vi "Result.Generate Xlink Overall Result.vi"(10 "Measurements":T2[](array[typedef]) {"Status" items=["LOG", "PASS", "FAIL", "ERROR"]}, 11 "Result":T4) -> (2 "PASS":bool, 3 "Measurement":T1)   [LabVIEW 2018]
uses:
  Result XML/TestResult.Symptom.ctl
  Result XML/TestResult.Symptom.State.ctl
  Result.Measurement Item.ctl
  Result.Measurement and Attribute Item Status.ctl
  Result.Factory Logix XLink Adapter, Measurement Item.ctl
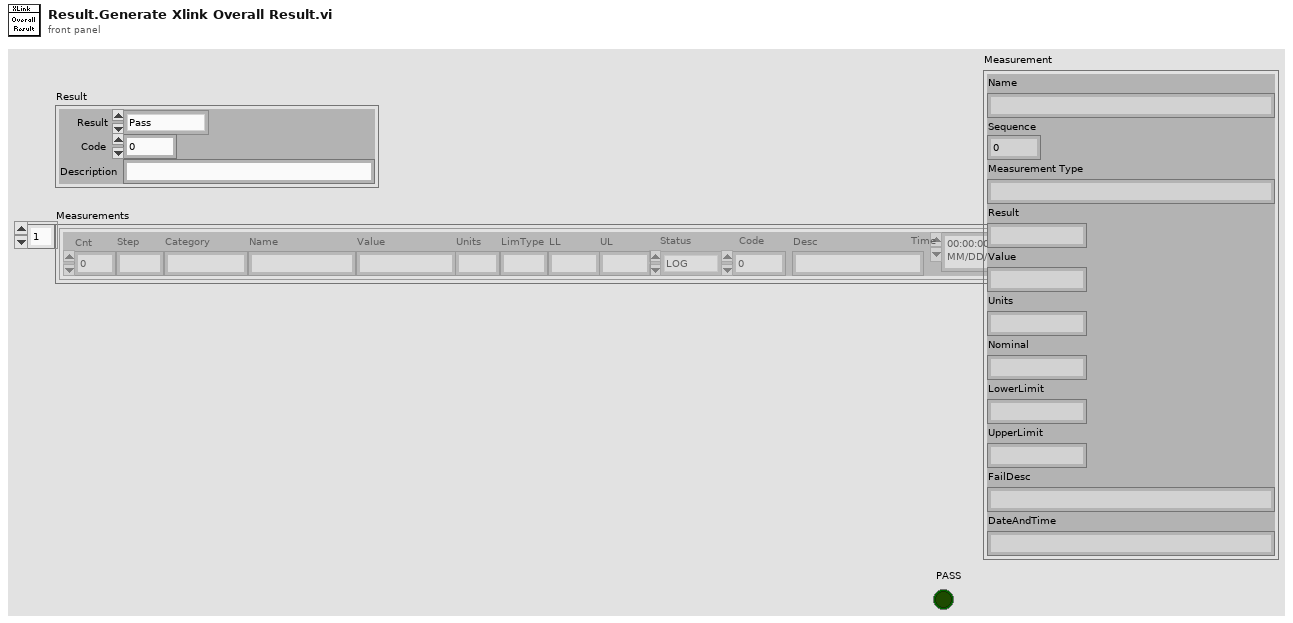
[diagram p1: front panel]
types:
  T1 = typedef "Result.Factory Logix XLink Adapter, Measurement Item.ctl" = cluster{"Name":string, "Sequence":i32, "Measurement Type":string, "Result":string, "Value":string, "Units":string, "Nominal":string, "LowerLimit":string, "UpperLimit":string, "FailDesc":string, "DateAndTime":string}
  T2 = typedef "Result.Measurement Item.ctl" = cluster{"Cnt":i32, "Step":string, "Category":string, "Name":string, "Value":string, "Units":string, "LimType":string, "LL":string, "UL":string, "Status":T3, "Code":i32, "Desc":string, "Time":timestamp}
  T3 = typedef "Result.Measurement and Attribute Item Status.ctl" = i32
  T4 = typedef "TestResult.Symptom.ctl" = cluster{"Result":T5, "Code":i32, "Description":string}
  T5 = typedef "TestResult.Symptom.State.ctl" = enum16{"Pass", "Fail", "Error", "Aborted", "Completed", "Logged"}
  T6 = cluster{"Pass":bool, "Code":string, "Name":string, "Meas":T1}
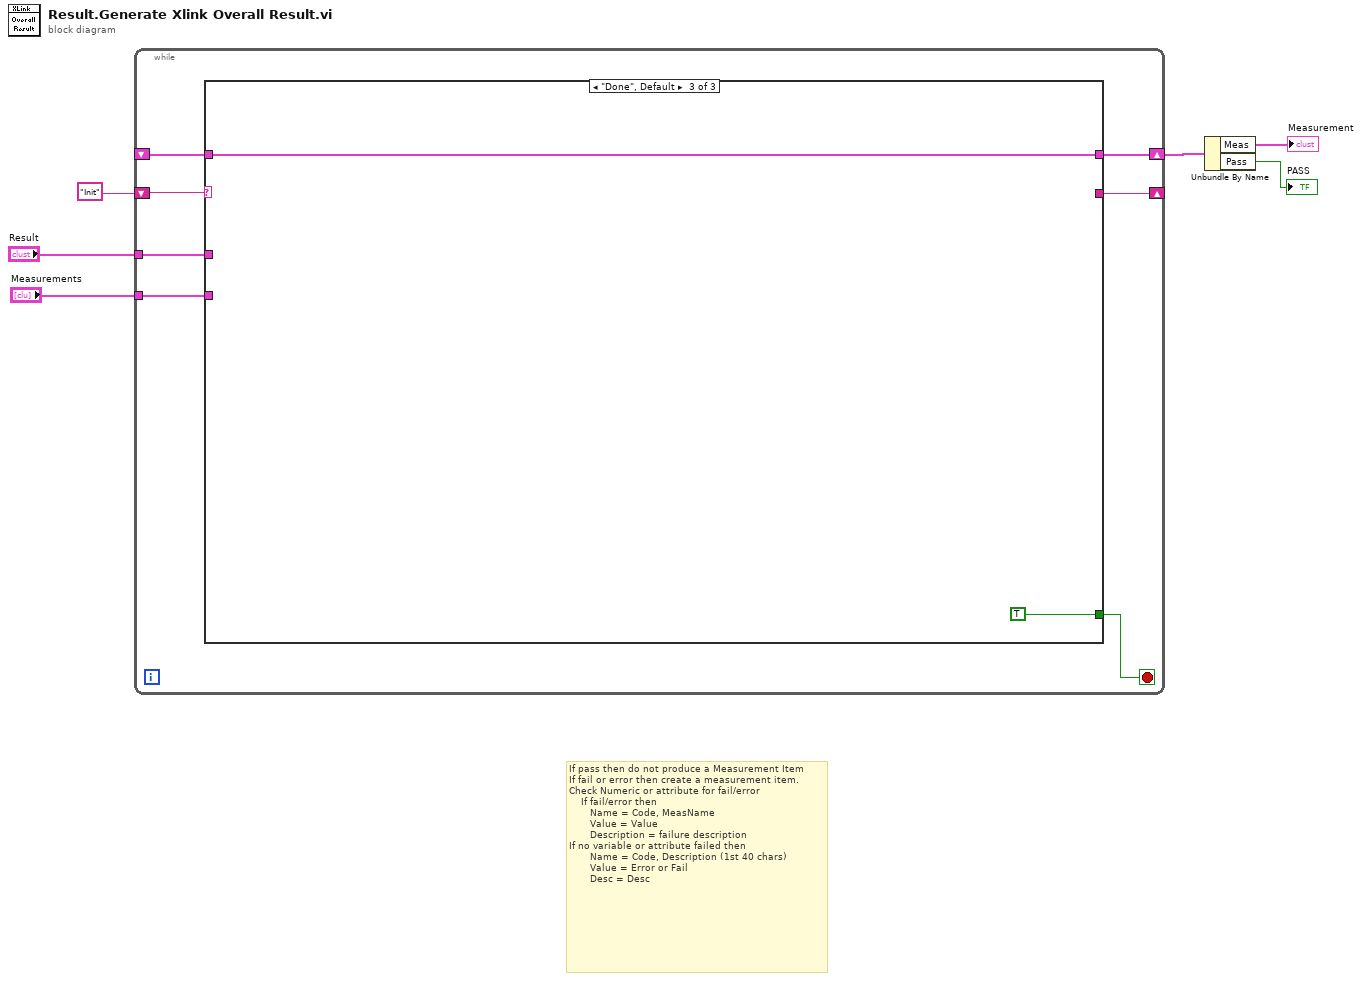
[diagram p0: block diagram]
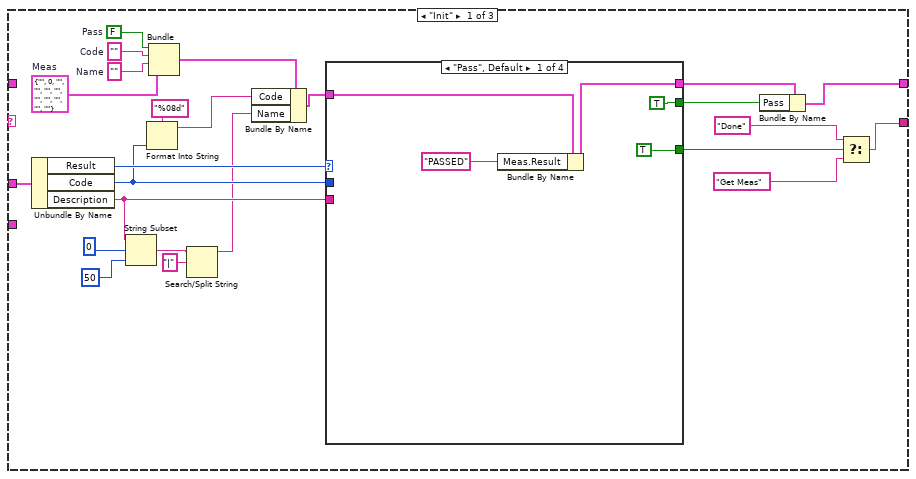
[diagram p2: hidden frame]
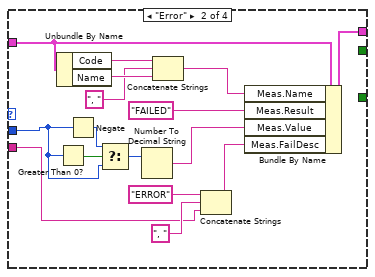
[diagram p3: hidden frame]
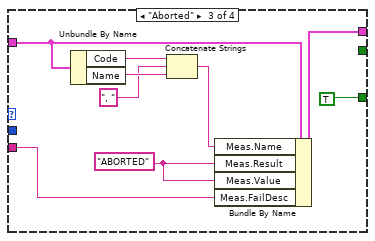
[diagram p4: hidden frame]
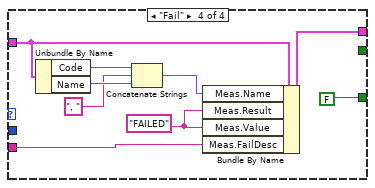
[diagram p5: hidden frame]
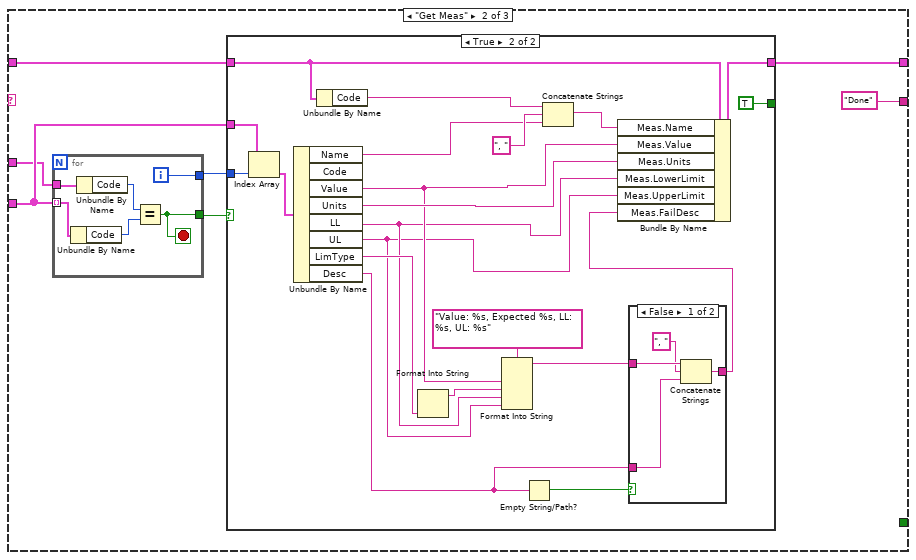
[diagram p6: hidden frame]
diagram:
  # "If pass then do not produce a Measurement Item\nIf fail or error then create a measurement item.\nCheck Numeric or attribute for fail/error\n    If fail/error then\n       Name = Code, MeasName\n       Value = Value\n       Description = failure description\nIf no variable or attribute failed then\n       Name = Code, Description (1st 40 chars)\n       Value = Error or Fail\n       Desc = Desc"
  n1 = while {
    shift-right: [w11] -> w3
    shift-left: _ -> [w13]
    shift-right: [w10] -> _
    shift-left: "Init" -> [w12]
    tunnel: "Result" -> [w8]
    tunnel: "Measurements" -> [w7]
    stop <- w9 stop-if-true
    n2 = case shown="\"Done\", Default" w12 {
      tunnel: w13 -> [_ w81 w117]
      tunnel: [w16 w80 w117] -> w11
      tunnel: [w35 "Done" _] -> w10
      tunnel: [_ _ TRUE] -> w9
      tunnel: w8 -> [w34 w78 _]
      tunnel: w7 -> [_ w82 _]
      frame "Init" {
        w18 = FALSE  # Pass
        w24 = ""  # Name
        w25 = ""  # Code
        w23 = T1 {"Name"="", "Sequence"=0, "Measurement Type"="", "Result"="", "Value"="", "Units"="", "Nominal"="", "LowerLimit"="", "UpperLimit"="", "FailDesc"="", "DateAndTime"=""}  # Meas
        n3 = Unbundle By Name(w34) -> ("Result"=w33:T5, "Code"=w26:i32, "Description"=w28:string)
        n4 = String Subset(string=w28, offset (0)=0, length (rest)=50 ("length (rest)")) -> (substring=w29:string)
        n5 = Format Into String(format string="%08d", w26) -> (resulting string=w20:string)  [unwired: 2 in, 1 out]
        n6 = Bundle("Pass"=w18, "Code"=w25, "Name"=w24, "Meas"=w23) -> (w22:T6)  [unwired: 1 in]
        n7 = Search/Split String(string=w29, search string/char (-)="|") -> (substring before match=w19:string)  [unwired: 1 in, 2 out]
        n8 = Bundle By Name(cluster=w22, "Code"=w20, "Name"=w19) -> (w21:T6)
        n9 = case shown="\"Pass\", Default" w33 {
          tunnel: w21 -> [w41 w47 w60 w69]
          tunnel: w26 -> [_ w52 _ _]
          tunnel: w28 -> [_ w49 w64 w73]
          tunnel: [w40 w58 w67 w76] -> w17
          tunnel: [TRUE _ TRUE FALSE] -> w15
          tunnel: [TRUE _ _ _] -> w14
          frame "Pass", Default {
            n10 = Bundle By Name(cluster=w41, "Meas.Result"="PASSED" ("Result")) -> (w40:T6)
          }
          frame "Error" {
            n11 = Unbundle By Name(w47) -> ("Code"=w46:string, "Name"=w45:string)
            n12 = Greater Than 0?(x=w52) -> (x > 0?=w54:bool)
            n13 = Negate(x=w52) -> (-x=w55:i32)
            n14 = Select(t=w55, s=w54, f=w52) -> (s? t:f=w51:i32)
            n15 = Number To Decimal String(number=w51) -> (decimal integer string=w48:string)  [unwired: 1 in]
            n16 = Concatenate Strings(w46, ", ", w45) -> (w43:string)
            n17 = Concatenate Strings("ERROR" ("Result"), ", ", w49) -> (w56:string)
            n18 = Bundle By Name(cluster=w47, "Meas.Name"=w43, "Meas.Result"="FAILED" ("Result"), "Meas.Value"=w48, "Meas.FailDesc"=w56) -> (w58:T6)
          }
          frame "Aborted" {
            w65 = "ABORTED" ("Result")
            n19 = Unbundle By Name(w60) -> ("Code"=w63:string, "Name"=w62:string)
            n20 = Concatenate Strings(w63, ", ", w62) -> (w59:string)
            n21 = Bundle By Name(cluster=w60, "Meas.Name"=w59, "Meas.Result"=w65, "Meas.Value"=w65, "Meas.FailDesc"=w64) -> (w67:T6)
          }
          frame "Fail" {
            w74 = "FAILED" ("Result")
            n22 = Unbundle By Name(w69) -> ("Code"=w72:string, "Name"=w71:string)
            n23 = Concatenate Strings(w72, ", ", w71) -> (w68:string)
            n24 = Bundle By Name(cluster=w69, "Meas.Name"=w68, "Meas.Result"=w74, "Meas.Value"=w74, "Meas.FailDesc"=w73) -> (w76:T6)
          }
        }
        n25 = Bundle By Name(cluster=w17, "Pass"=w14) -> (w16:T6)
        n26 = Select(t="Done", s=w15, f="Get Meas") -> (s? t:f=w35:string)
      }
      frame "Get Meas" {
        n27 = for {
          tunnel: w82 -> [w116] mode=indexing
          tunnel: [w115] -> w79
          tunnel: [w114] -> w83
          tunnel: w78 -> [w112]
          i -> [w114]
          stop <- w115 stop-if-true
          n28 = Unbundle By Name(w116) -> ("Code"=w113:i32)
          n29 = Unbundle By Name(w112) -> ("Code"=w111:i32)
          n30 = Equal?(x=w111, y=w113) -> (x = y?=w115:bool)
        }
        n31 = case shown="True" w79 {
          tunnel: w83 -> [_ w105]
          tunnel: w82 -> [_ w104]
          tunnel: w81 -> [w84 w89]
          tunnel: [w84 w101] -> w80
          tunnel: [_ TRUE] -> _
          frame False {
          }
          frame True {
            n32 = Index Array(array=w104, index=w105) -> (element=w103:T2)
            n33 = Unbundle By Name(w103) -> ("Name"=w90:string, "Value"=w87:string, "Units"=w99:string, "LL"=w86:string, "UL"=w85:string, "LimType"=w95:string, "Desc"=w94:string)  [unwired: 1 out]
            n34 = Unbundle By Name(w89) -> ("Code"=w88:string)
            n35 = Format Into String(w95) -> (resulting string=w96:string)  [unwired: 3 in, 1 out]
            n36 = Format Into String(format string="Value: %s, Expected %s, LL: %s, UL: %s", w87, w96, w86, w85) -> (resulting string=w97:string)  [unwired: 2 in, 1 out]
            n37 = Empty String/Path?(string/path=w94) -> (empty?=w93:bool)
            n38 = Concatenate Strings(w88, ", ", w90) -> (w100:string)
            n39 = case shown="False" w93 {
              tunnel: w97 -> [w109 w110]
              tunnel: w94 -> [w108 _]
              tunnel: [w106 w110] -> w92
              frame False {
                n40 = Concatenate Strings(w109, ", ", w108) -> (w106:string)
              }
              frame True {
              }
            }
            n41 = Bundle By Name(cluster=w89, "Meas.Name"=w100, "Meas.Value"=w87, "Meas.Units"=w99, "Meas.LowerLimit"=w86, "Meas.UpperLimit"=w85, "Meas.FailDesc"=w92) -> (w101:T6)
          }
        }
      }
      frame "Done", Default {
      }
    }
  }
  n42 = Unbundle By Name(w3) -> ("Meas"=→"Measurement":T1, "Pass"=→"PASS":bool)
